vi "Dashboard Main.vi"() -> ()   [LabVIEW 2016]
uses:
  <vilib>/Utility/miscctls.llb/LVRowAndColumnTypeDef.ctl
  <vilib>/event_ctls.llb/eventvkey.ctl
  <vilib>/Rock Robotics/Network Tables/NT Read Numeric Array.vi
  <vilib>/Rock Robotics/Network Tables/NT Read Boolean.vi
  <vilib>/Rock Robotics/Network Tables/NT Write String Array.vi
  <vilib>/Rock Robotics/Network Tables/NT Write Numeric Array.vi
  <vilib>/Rock Robotics/WPI/Dashboard/WPI_DashboardLogging Global.vi
panel:
  out "JS1 Z":dbl(slide) scale=-1.0..1.0 scale format="%#_2e"
  out "JS1 Graph":cluster{"X":dbl, "Y":dbl}[](graph)
  out "JS1 Buttons":T1
  out "JS2 Z":dbl(slide) scale=-1.0..1.0 scale format="%#_2e"
  out "JS2 Graph":cluster{"X":dbl, "Y":dbl}[](graph)
  out "JS2 Buttons":T1
  in  "Camera Settings Right":T2={"Frame Rate"=30, "Compression"=30, "Size"=1, "DB Camera Config"=FALSE} {"Frame Rate" scale=1.0..30.0; "Compression" scale=100.0..-1.0; "Size" items=["640x480", "320x240", "160x120"]}
  in  "Camera Name Right":string(combo)="No Camera Selection"
  out "Camera Info":cluster{"Mbps LED":bool, "Mbps":dbl, "fps":dbl} {"fps" format="%#.1g"; "Mbps" format="%#.1g"}
  in  "Camera Settings":T2={"Frame Rate"=30, "Compression"=30, "Size"=1, "DB Camera Config"=FALSE} {"Frame Rate" scale=1.0..30.0; "Compression" scale=100.0..-1.0; "Size" items=["640x480", "320x240", "160x120"]}
  in  "TCP":refnum<k5>
  in  "Rec Mode":enum32{"Stop", "Record", "Playback"}(radio)
  out "Robot IP":string
  out "Image Message":string="Timeout in Camera Communications"
  in  "Dashboard Tab":T3(tab)
  out "Gyro Angle":dbl
  in  "Refresh Auto":bool
  out "NT Connection":bool
  out "MotorChart R":cluster{"Numeric":dbl, "Numeric":dbl}(graph)
  out "MotorChart L":cluster{"Numeric":dbl, "Numeric":dbl}(graph)
  out "MotorSliders R":cluster{"MotorSlide1":dbl, "MotorSlide2":dbl} {"MotorSlide2" scale=-1.0..1.0 scale format="%#_2e"; "MotorSlide1" scale=-1.0..1.0 scale format="%#_2e"}
  out "MotorSliders L":cluster{"MotorSlide1":dbl, "MotorSlide2":dbl} {"MotorSlide2" scale=-1.0..1.0 scale format="%#_2e"; "MotorSlide1" scale=-1.0..1.0 scale format="%#_2e"}
  out "Gyro":dbl(knob) scale=0.0..360.0
  out "Mode":T4(ring)=enum."Auto Disabled"
  out "Ball Intake Speed":dbl(slide) scale=0.0..1.0
  out "Shooter Speed":dbl(slide) scale=0.0..1.0
  in  "Auto Routines":string(combo)
  out "Auto Cmd":string
  out "Auto Arg":string
  out "Climber":bool
  out "IMU AHRS":cluster{"Pitch":dbl, "Roll":dbl, "Yaw":dbl}
  out "IMU Angle":cluster{"X":dbl, "Y":dbl, "Z":dbl}
  out "Front Left Encoder":dbl
  out "Front Right Encoder":dbl
  out "Back Right Encoder":dbl
  out "Back Left Encoder":dbl
  out "Camera Image Right":T5(plugin-control)
  in  "DB/String 9":string
  in  "DB/String 8":string
  in  "DB/String 7":string
  in  "DB/String 6":string
  in  "DB/String 5":string
  in  "DB/String 4":string
  in  "DB/String 3":string
  in  "DB/String 2":string
  in  "DB/String 1":string
  in  "DB/String 0":string
  in  "DB/Slider 0":dbl(slide) scale=0.0..5.0
  in  "DB/Slider 1":dbl(slide) scale=0.0..5.0
  in  "DB/Slider 2":dbl(slide) scale=0.0..5.0
  in  "DB/Slider 3":dbl(slide) scale=0.0..5.0
  out "DB/LED 3":bool
  out "DB/LED 2":bool
  out "DB/LED 1":bool
  out "DB/LED 0":bool
  in  "DB/Button 3":bool
  in  "DB/Button 2":bool
  in  "DB/Button 1":bool
  in  "DB/Button 0":bool caption="New Name"
  in  "Test Slider":dbl(slide) scale=0.0..100.0 scale format="%#_3g"
  in  "On/Off":bool caption="Solenoid"
  in  "Test Name":u16(ring) items=["Select the test to run..."]
  in  "Test Tree":string(tree)
  in  "Motor":cluster{"Value":dbl, "Enable":bool} {"Value" scale=-1.0..1.0 scale format="%#_3g"}
  out "Progress":T6 {"Test Progress" scale=0.0..100.0}
  in  "Rev/Fwd":cluster{"Forward":bool, "Reverse":bool}
  in  "Test Ring":u16(ring) items=["Monochrome", "Color"]
  out "Cmd Status":string
  in  "Execute Command":bool
  in  "Command Params":string[][](table)
  in  "Command Selection":i32(listbox)
  in  "CheckList":i32(listbox)
  out "Tree":string(tree)
  out "Camera Image":T5(plugin-control)
  out "Background":bool
  in  "Camera Name":string(combo)="No Camera Selection"
  # "Joysticks"
  # "HW"
  # "HW"
  # "Drive Motors"
  # "Front"
  # "Right"
  # "Left"
  # "Back"
  # "This tab is a great place for autonomous settings and robot-specific values.\nPlace controls and indicators inside this tab and match name to\nDashboard Variables on robot. You can also delete this comment."
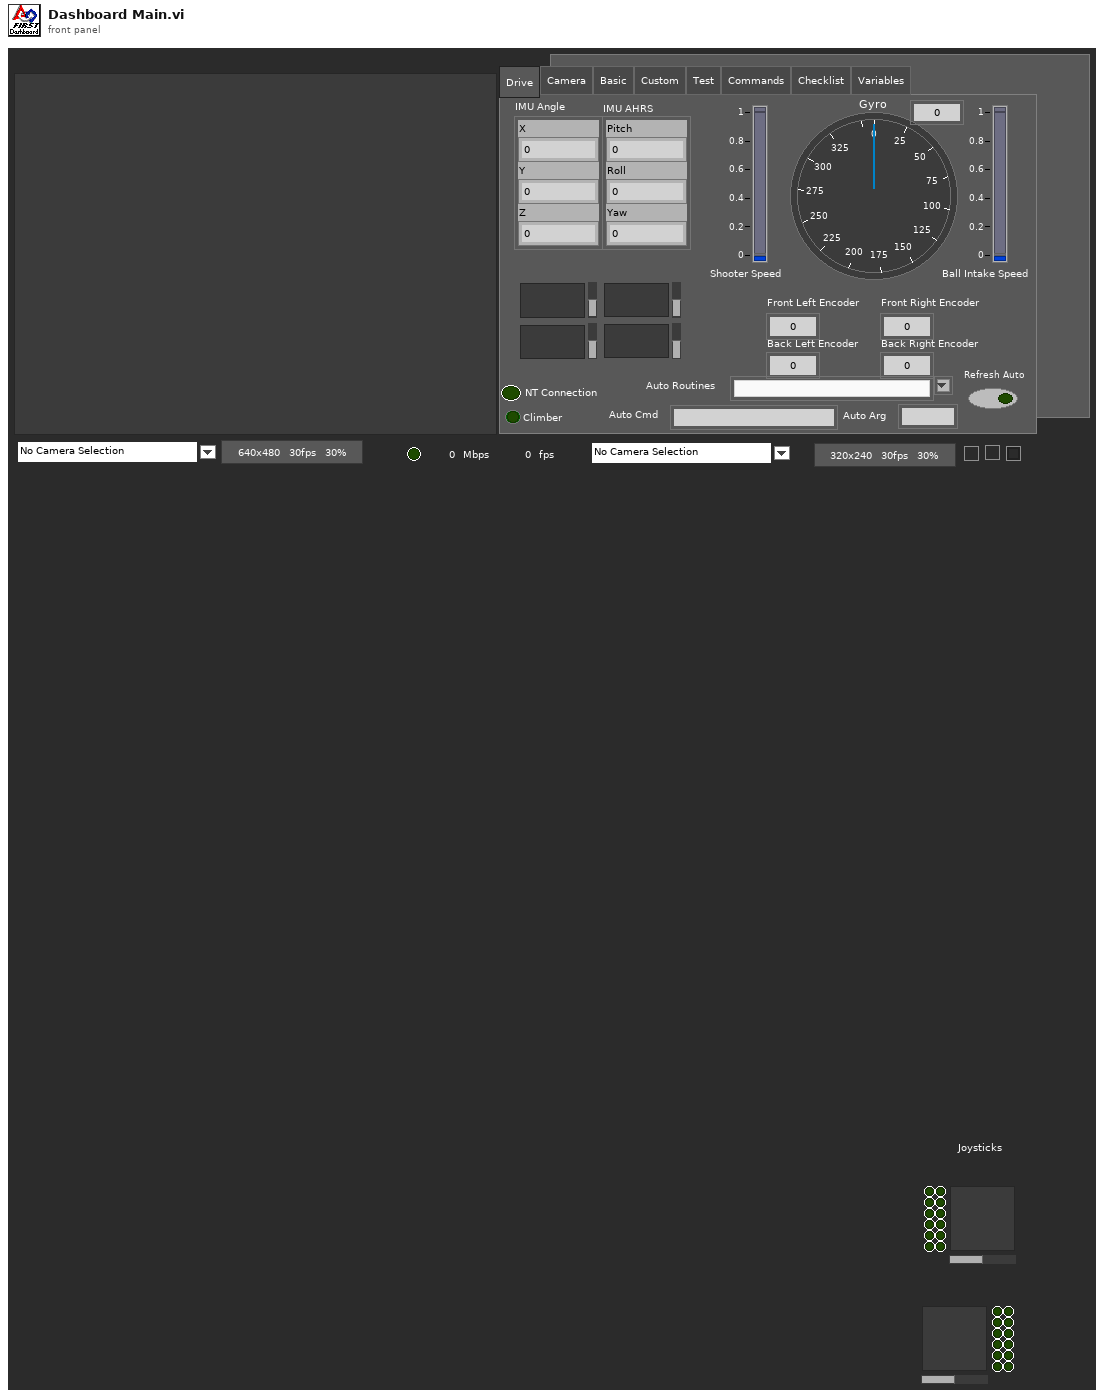
[diagram p1: front panel]
types:
  T1 = cluster{bool, bool, bool, bool, bool, bool, bool, bool, bool, bool, bool, bool}
  T2 = cluster{"Frame Rate":i32, "Compression":i32, "Size":u16, "DB Camera Config":bool}
  T3 = enum32{"Drive", "Camera", "Basic", "Custom", "Test", "Commands", "Checklist", "Variables"}
  T4 = enum8{"Tele-Op Disabled", "Tele-Op Enabled", "Auto Disabled", "Auto Enabled", "Test Disabled", "Test Enabled", "Disconnected", "No Code", "E-Stop"}
  T5 = typedef "IMAQ Image.ctl" = refnum<image>
  T6 = cluster{"Test Progress":u8, "Test Progress Text":string}
  T7 = typedef "Image Type" = u32
  T8 = cluster{"IDs":cluster{"RPC field ID":u16, "Unique ID":u16}, "String":string}
  T9 = enum32{"Drive", "Basic", "Custom", "Test", "Checklist", "Variables"}
  T10 = cluster{"Error Strings":string, "Disable Counts":cluster{u16, u16}, "Rail Faults":cluster{u16, u16, u16}, "Robot IP":string, "DB Mode":u8, "Event Info":cluster{"Name":string, "Type":u8, "Number":u16, "Replay":u8}}
  T11 = cluster{"Storage":cluster{"Disk Free":u64, "RAM Block":u32, "RAM free":u32}, "CPU Utilization":cluster{"CPU % ISR":sgl, "CPU % Time Crit":sgl, "CPU % Timed Str":sgl, "CPU % High":sgl, "CPU % Above":sgl, "CPU % Normal":sgl, "CPU % Low":sgl}, "CAN":cluster{"% Bus Utilization":sgl, "Bus Off Cnt":u32, "TX_FIFO Full Cnt":u32, "Receive Error Cnt":u8, "Transmit Error Cnt":u8}, "HID":cluster{"HID Outputs":u32, "Rumble Low":u16, "Rumble High":u16}[]}
  T12 = cluster{"Status bits":cluster{"Test Mode":bool, "Autonomous":bool, "Enabled":bool, "Code Start":bool, "Brownout":bool, "Reserved 2":bool, "Reserved 3":bool, "E-Stop":bool}, "Code Trace":cluster{"Disabled":bool, "TeleOp":bool, "Auto":bool, "Test":bool}, "Controller Type":enum16{"unknown", "cRIO", "roboRio"}, "Code?":enum16{"unknown", "noCode", "code"}, "Battery V":dbl}
  T13 = cluster{"Control Bits":cluster{"TestMode":bool, "Autonomous":bool, "Enabled":bool, "FMS Present":bool, bool, bool, bool, "E-Stop":bool}, "Team Station ":u8, "Countdown":sgl, "Joystick Values":cluster{"Axes":dbl[], "Buttons":bool[], "POVs":i16[]}[]}
  T14 = cluster{"Axes":dbl[], "Buttons":bool[], "POVs":i16[]}[]
  T15 = cluster{"Numeric Array[0]":dbl, "Numeric Array[1]":dbl, "Numeric Array[2]":dbl, "Numeric Array[3]":dbl, "Numeric Array[4]":dbl, "Numeric Array[5]":dbl, "Numeric Array[6]":dbl, "Numeric Array[7]":dbl, "Numeric Array[8]":dbl}
  T16 = cluster{"Axes":dbl[], "Buttons":bool[], "POVs":i16[]}
  T17 = cluster{"Buttons[0]":bool, "Buttons[1]":bool, "Buttons[2]":bool, "Buttons[3]":bool, "Buttons[4]":bool, "Buttons[5]":bool, "Buttons[6]":bool, "Buttons[7]":bool, "Buttons[8]":bool, "Buttons[9]":bool, "Buttons[10]":bool, "Buttons[11]":bool}
  T18 = cluster{"Camera Image":refnum<vi>, "Dashboard Tab":refnum<vi>, "Background":refnum<vi>, "Rec Mode":refnum<vi>, "Test Slider":refnum<vi>, "On/Off ":refnum<vi>, "Test Ring":refnum<vi>, "Rev/Fwd":refnum<vi>, "Test Name":refnum<vi>, "Motor":refnum<vi>, "Progress":refnum<vi>, "CheckList":refnum<vi>, "Tree":refnum<vi>, "Test Tree":refnum<vi>, "Command Params":refnum<vi>, "Command Selection":refnum<vi>, "Execute Command":refnum<vi>, "Cmd Status":refnum<vi>, "Camera Settings":refnum<vi>, "Camera Name":refnum<vi>, "Camera Info":refnum<vi>, "Camera Settings Right":refnum<vi>, "Camera Name Right":refnum<vi>, "Camera Image Right":refnum<vi>}
  T19 = cluster{"Operation":enum16{"Update", "Clear"}, "Color Box":u32}[]
  T20 = typedef "eventvkey.ctl" = enum16{"ASCII", "Enter", "Return", "Shift", "Ctrl", "Alt", "Cmd", "Opt", "Caps", "NumLock", "Clear", "Break", "Up", "Down", "Left", "Right", "Insert", "Delete", "Home", "End", "PageUp", "PageDown", "Escape", "Help", "Pause", "ScrollLock", "F1", "F2", "F3", "F4", "F5", "F6", "F7", "F8", "F9", "F10", "F11", "F12", "F13", "F14", "F15", "F16", "F17", "F18", "F19", "F20", "F21", "F22", "F23", "F24", "Play", "VolumeUp", "VolumeDown", "Mute", "Two Byte Char"}
  T21 = cluster{"Image Size":bool, "Image Type":bool, "Pixel Value":bool, "ROI Information":bool, "Zoom Factor":bool}
  T22 = cluster{"Operation":enum16{"Update", "Clear"}, "Color Box":u32}
  T23 = typedef "LVRowAndColumnTypeDef.ctl" = cluster{"Row":i32, "Column":i32}
  T24 = cluster{"Shift":bool, "Ctrl":bool, "Alt":bool, "Cmd":bool, "Opt":bool}
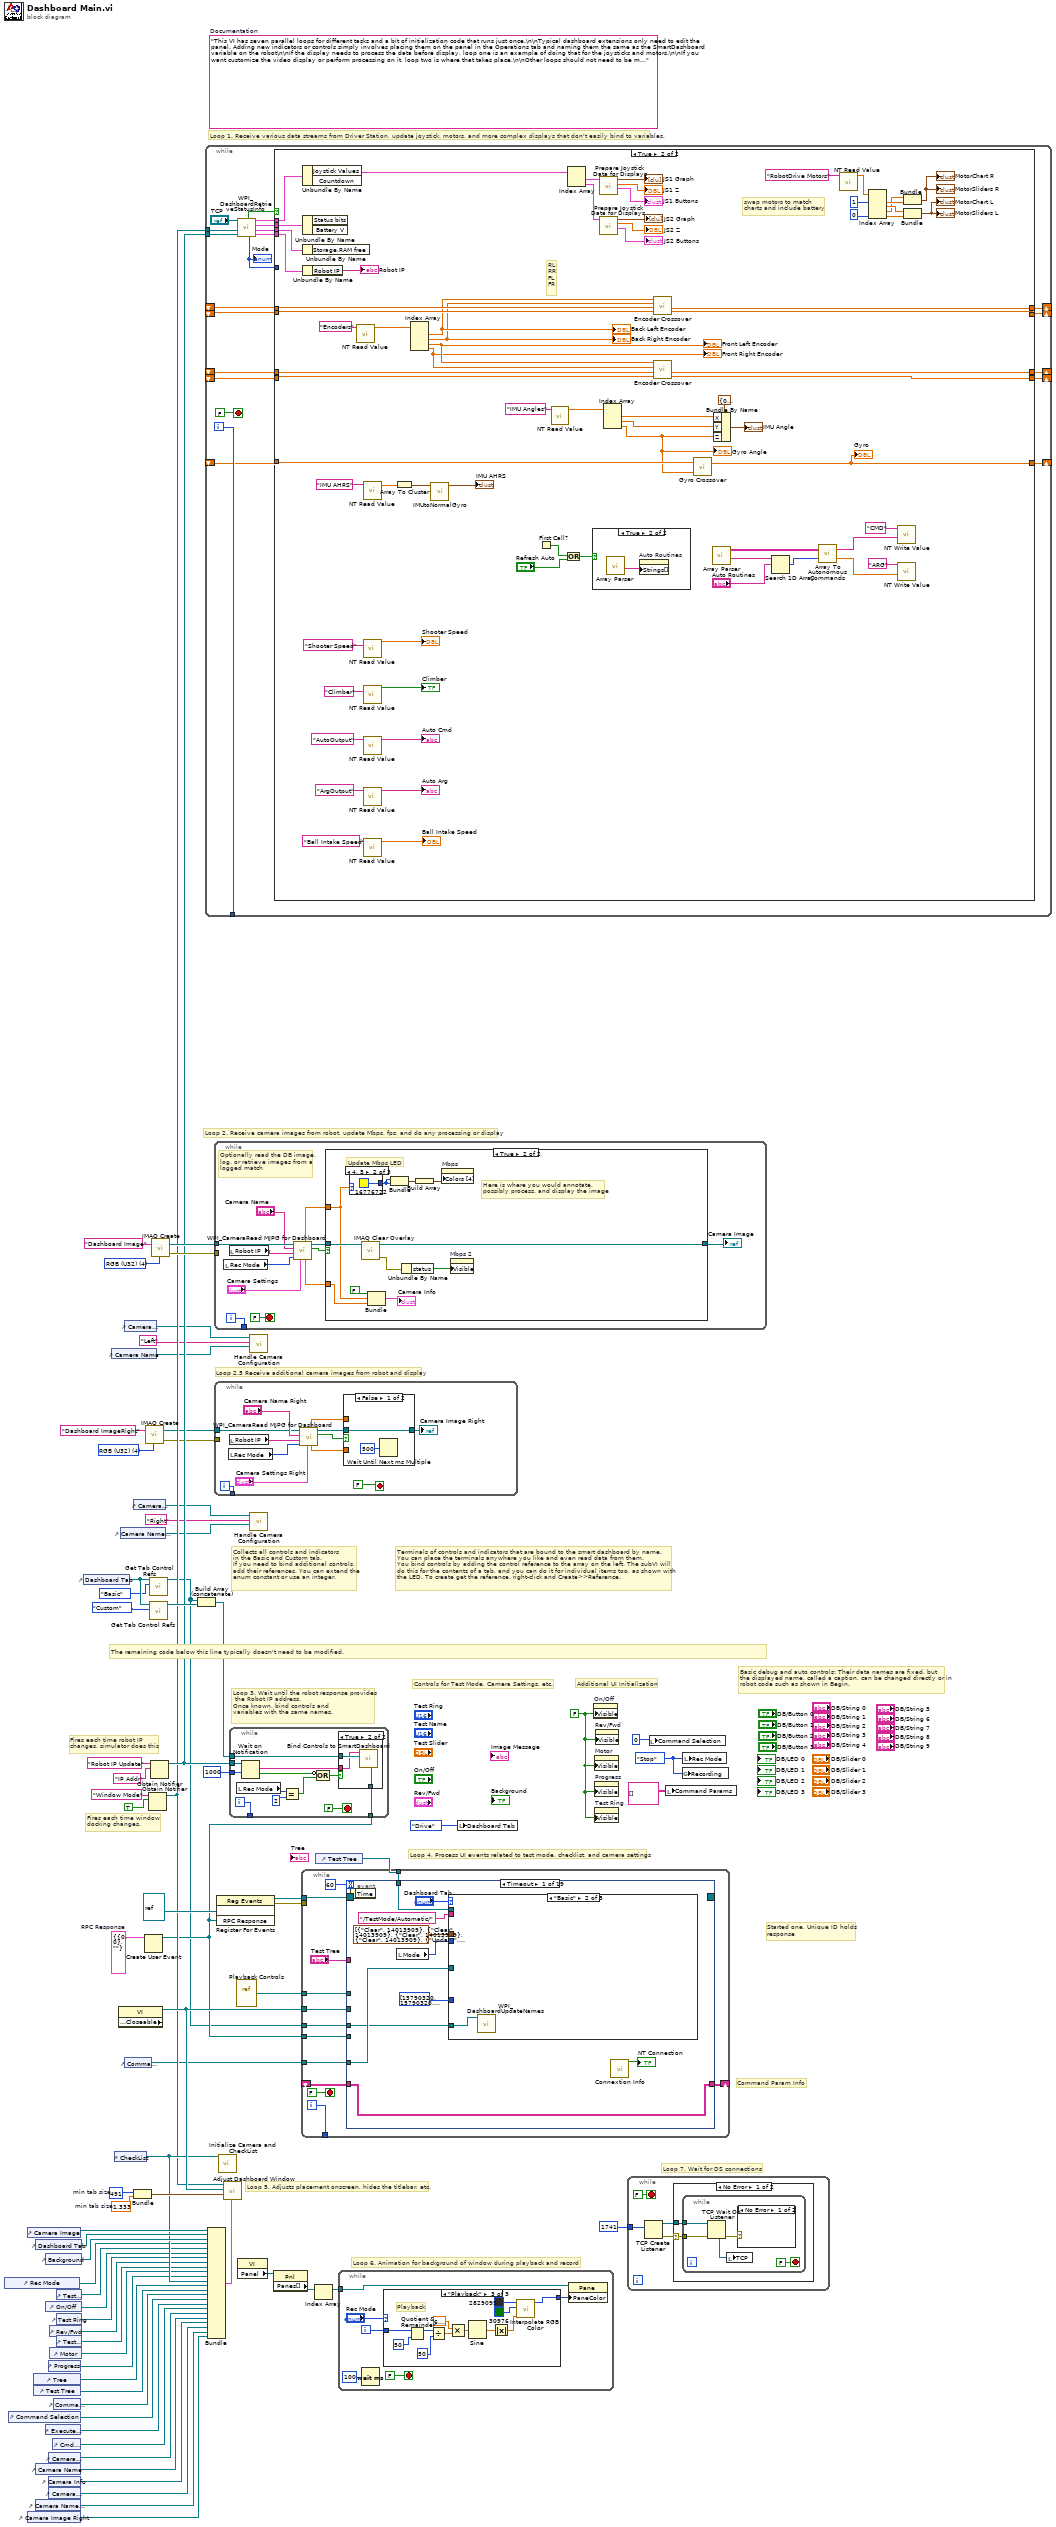
[diagram p0: block diagram]
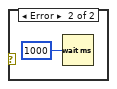
[diagram p3: hidden frame]
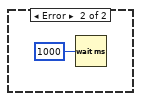
[diagram p4: hidden frame]
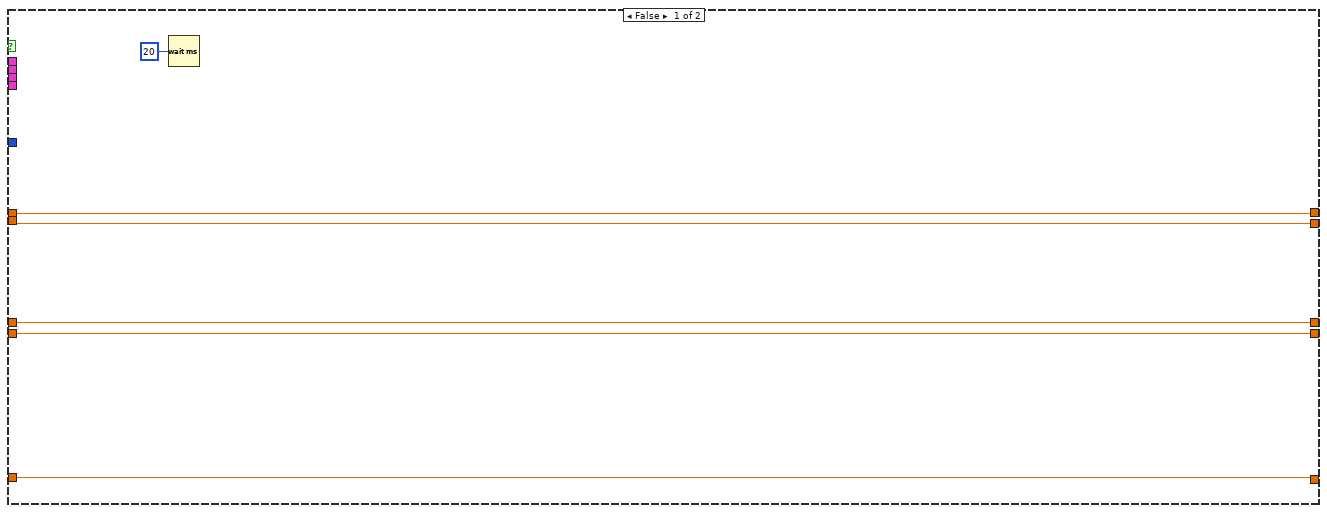
[diagram p5: hidden frame]
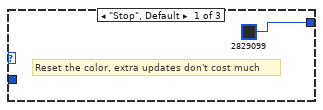
[diagram p7: hidden frame]
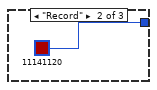
[diagram p8: hidden frame]
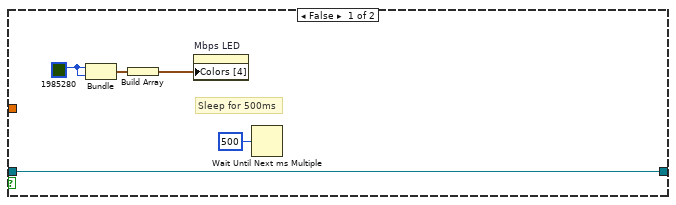
[diagram p10: hidden frame]
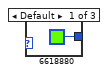
[diagram p11: hidden frame]
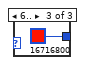
[diagram p12: hidden frame]
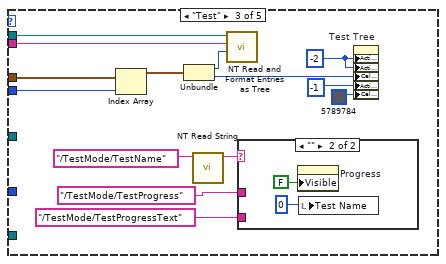
[diagram p14: hidden frame]
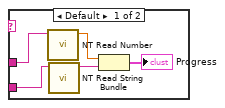
[diagram p15: hidden frame]
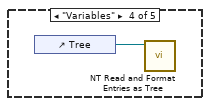
[diagram p16: hidden frame]
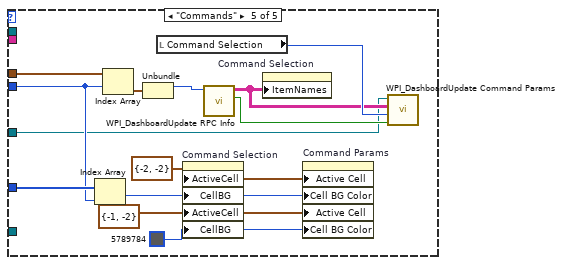
[diagram p17: hidden frame]
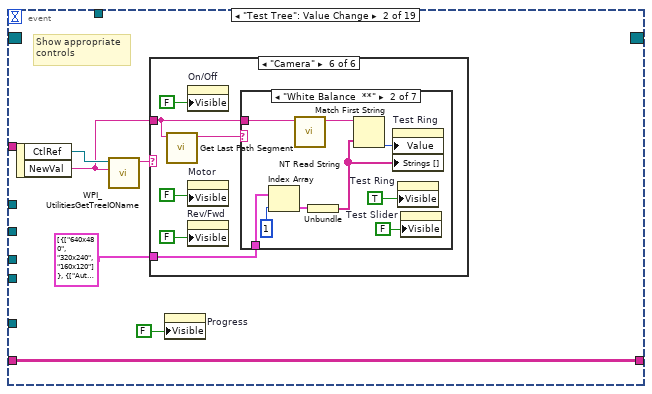
[diagram p18: hidden frame]
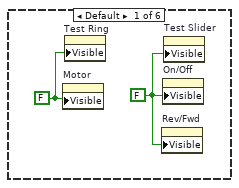
[diagram p19: hidden frame]
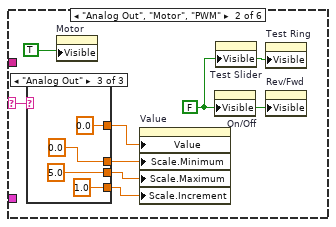
[diagram p20: hidden frame]
diagram:
  w10 = T7 4 items=["Grayscale (U8)", "Grayscale (I16)", "Grayscale (SGL)", "Complex (CSG)", "RGB (U32)", "HSL (U32)", "RGB (U64)"] ("Image Type")
  w24 = T8 {"IDs"={"RPC field ID"=0, "Unique ID"=0}, "String"=""}  # RPC Response
  w49 = 491  # min tab size
  w48 = 1.333  # min tab size
  w56 = enum32{"Stop", "Record", "Playback"}."Stop" ("Rec Mode")
  w31 = FALSE ("Visible")
  (unwired) "This VI has seven parallel loops for different tasks and a bit of initialization code that runs just once.\n\nTypical dashboard extensions only need to edit the panel. Adding new indicators or controls simply involves placing them on the panel in the Operations tab and naming them the same as the SmartDashboard variable on the robot\n\nIf the display needs to process the data before display, loop one is an example of doing that for the joysticks and motors.\n\nIf you want customize the video display or perform processing on it, loop two is where that takes place.\n\nOther loops should not need to be modified. They are pretty standard, and document the task they perform."  # Documentation
  w73 = T7 4 items=["Grayscale (U8)", "Grayscale (I16)", "Grayscale (SGL)", "Complex (CSG)", "RGB (U32)", "HSL (U32)", "RGB (U64)"] ("Image Type")
  # "Loop 2.5 Receive additional camera images from robot and display"
  # "Command Param Info"
  # "Started one, Unique ID holds\nresponse"
  # "Loop 7. Wait for DS connections"
  # "Basic debug and auto controls: Their data names are fixed, but\nthe displayed name, called a caption, can be changed directly or in\nrobot code such as shown in Begin."
  # "Controls for Test Mode, Camera Settings, etc."
  # "Additional UI Initialization"
  # "Loop 6. Animation for background of window during playback and record"
  # "Fires each time robot IP\nchanges, simulator does this"
  # "Fires each time window\ndocking changes."
  # "Collects all controls and indicators\nin the Basic and Custom tab.\nIf you need to bind additional controls,\nadd their references. You can extend the\nenum constant or use an integer."
  # "The remaining code below this line typically doesn't need to be modified."
  # "Loop 4. Process UI events related to test mode, checklist, and camera settings"
  # "Terminals of controls and indicators that are bound to the smart dashboard by name.\nYou can place the terminals anywhere you like and even read data from them.\nYou bind controls by adding the control reference to the array on the left. The subVI will\ndo this for the contents of a tab, and you can do it for individual items too, as shown with\nthe LED. To create get the reference, right-click and Create>>Reference."
  # "Loop 3. Wait until the robot response provides\n the Robot IP address.\nOnce known, bind controls and\nvariables with the same names."
  # "Loop 5. Adjusts placement onscreen, hides the titlebar, etc."
  # "Loop 1. Receive various data streams from Driver Station, update joystick, motors, and more complex displays that don't easily bind to variables."
  # "Loop 2. Receive camera images from robot, update Mbps, fps, and do any processing or display"
  n1 = control-ref of="Rec Mode"() -> (w37:refnum<vi>)
  n2 = control-ref of="Command Selection"() -> (w23:refnum<vi>)
  n3 = control-ref of="Camera Image Right"() -> (w1:refnum<vi>)
  n4 = control-ref of="Camera Image"() -> (w51:refnum<vi>)
  n5 = control-ref of="Tree"() -> (w41:refnum<vi>)
  n6 = control-ref of="Test Tree"() -> (w40:refnum<vi>)
  n7 = control-ref of="Dashboard Tab"() -> (w50:refnum<vi>)
  n8 = control-ref of="Camera Name"() -> (w14:refnum<vi>)
  n9 = control-ref of="Camera Name Right"() -> (w2:refnum<vi>)
  n10 = control-ref of="Execute Command"() -> (w25:refnum<vi>)
  n11 = control-ref of="Background"() -> (w46:refnum<vi>)
  n12 = control-ref of="On/Off"() -> (w35:refnum<vi>)
  n13 = control-ref of="Progress"() -> (w32:refnum<vi>)
  n14 = control-ref of="Camera Settings"() -> (w15:refnum<vi>)
  n15 = control-ref of="Camera Info"() -> (w13:refnum<vi>)
  n16 = control-ref of="Camera Settings Right"() -> (w3:refnum<vi>)
  n17 = control-ref of="Rev/Fwd"() -> (w33:refnum<vi>)
  n18 = control-ref of="Motor"() -> (w38:refnum<vi>)
  n19 = control-ref of="Cmd Status"() -> (w19:refnum<vi>)
  n20 = control-ref of="Command Params"() -> (w26:refnum<vi>)
  n21 = control-ref of="Test Slider"() -> (w36:refnum<vi>)
  n22 = control-ref of="Test Ring"() -> (w34:refnum<vi>)
  n23 = control-ref of="Test Name"() -> (w39:refnum<vi>)
  n24 = control-ref of="Dashboard Tab"() -> (w54:refnum<vi>)
  n25 = control-ref of="Camera Name"() -> (w16:refnum<vi>)
  n26 = control-ref of="CheckList"() -> (w42:refnum<vi>)
  n27 = property class="VI" props=["Front Panel.Closeable"]() -> (reference out=w55:refnum<vi>)  [unwired: 2 in, 2 out]
  n28 = control-ref of="Camera Name Right"() -> (w6:refnum<vi>)
  n29 = control-ref of="Camera Settings"() -> (w17:refnum<vi>)
  n30 = control-ref of="Command Params"() -> (w18:refnum<vi>)
  n31 = control-ref of="Camera Settings Right"() -> (w7:refnum<vi>)
  n32 = Bundle("min tab size"=w49, "min tab size"=w48) -> (w47:cluster{"min tab size":i32, "min tab size":dbl})  [unwired: 1 in]
  n33 = Create User Event(user event datatype=w24) -> (user event=w20:refnum<user-event>)  [unwired: 1 in, 1 out]
  n34 = call "IMAQ Create"("Image Name"="Dashboard ImageRight", "Image Type"=w10) -> ("New Image"=w9:T5, "error out"=w8:errorcluster)  [unwired: 2 in, 1 out]
  n35 = Obtain Notifier(name (unnamed)="Window Mode", notification data type=TRUE) -> (notifier out=w29:refnum<notifier>)  [unwired: 2 in, 2 out]
  n36 = call <vilib>:"Get Tab Control Refs.vi"("Page Index"=T9."Basic" ("Dashboard Tab"), "TabControl in"=w54) -> ("ControlsOnPage"=w12:refnum<vi>[])  [unwired: 9 in]
  n37 = call <vilib>:"Get Tab Control Refs.vi"("Page Index"=T9."Custom" ("Dashboard Tab"), "TabControl in"=w54) -> ("ControlsOnPage"=w53:refnum<vi>[])  [unwired: 9 in]
  n38 = Obtain Notifier(name (unnamed)="Robot IP Update", notification data type="IP Addr" ("name (unnamed)")) -> (notifier out=w30:refnum<notifier>)  [unwired: 2 in, 2 out]
  n39 = call "IMAQ Create"("Image Name"="Dashboard Image", "Image Type"=w73) -> ("New Image"=w71:T5, "error out"=w70:errorcluster)  [unwired: 2 in, 1 out]
  n40 = Build Array (concatenate)(w12, w53) -> (w52:refnum<vi>[])
  n41 = while {
    tunnel: [w93] -> _
    tunnel: w30 -> [w87]
    tunnel: w29 -> [w84]
    shift-right: [w82] -> _
    shift-left: _ -> [w83]
    shift-right: [w80] -> _
    shift-left: _ -> [w81]
    shift-right: [w78] -> _
    shift-left: _ -> [w79]
    shift-right: [w74] -> _
    shift-left: _ -> [w75]
    shift-right: [w76] -> _
    shift-left: _ -> [w77]
    i -> [w93]
    stop <- FALSE stop-if-true
    n42 = call <vilib>:"WPI_DashboardRetrieveStatusInfo.vi"("Binding Refnum"=w87, "Window Mode Notifier"=w84, "TCP Cnx"="TCP") -> ("Power and Errors"=w88:T10, "Robot Metrics"=w91:T11, "Status Info"=w92:T12, "Control Info"=w89:T13, "Robot Mode"=w86:T4, "Process?"=w90:bool)  [unwired: 3 in]
    "Mode" <- w86
    n43 = case shown="True" w90 {
      tunnel: w92 -> [_ w172]
      tunnel: w91 -> [_ w171]
      tunnel: w89 -> [_ w170]
      tunnel: w88 -> [_ w169]
      tunnel: w86 -> [_ _]
      tunnel: [w98 w146] -> w82
      tunnel: [w97 w145] -> w80
      tunnel: w83 -> [w98 w144]
      tunnel: w81 -> [w97 w143]
      tunnel: w79 -> [w99 w142]
      tunnel: [w99 w102] -> w78
      tunnel: w77 -> [w96 w110]
      tunnel: [w96 w109] -> w76
      tunnel: w75 -> [w95 w108]
      tunnel: [w95 w107] -> w74
      frame False {
        n44 = Wait (ms)(milliseconds to wait=u32 20) -> ()  [unwired: 1 out]
      }
      frame True {
        # "RL\nRR\nFL\nFR"
        # "swap motors to match\ncharts and include battery"
        n45 = Unbundle By Name(w170) -> ("Joystick Values"=w160:T14)  [unwired: 1 out]
        n46 = Unbundle By Name(w172) -> ()  [unwired: 2 out]
        n47 = Unbundle By Name(w171) -> ()  [unwired: 1 out]
        n48 = Unbundle By Name(w169) -> ("Robot IP"=→"Robot IP":string)
        n49 = call-poly <vilib>:"NT Read Value.vi"("Name"="Encoders") -> ("Numeric Array"=w148:dbl[])  [unwired: 9 in, 1 out]
        n50 = call-poly <vilib>:"NT Read Value.vi"("Name"="Shooter Speed") -> ("Numeric"=→"Shooter Speed":dbl)  [unwired: 9 in, 1 out]
        n51 = call-poly <vilib>:"NT Read Value.vi"("Name"="Climber") -> ("Boolean"=→"Climber":bool)  [unwired: 9 in, 1 out]
        n52 = call-poly <vilib>:"NT Read Value.vi"("Name"="AutoOutput") -> ("String"=→"Auto Cmd":string)  [unwired: 9 in, 1 out]
        n53 = call-poly <vilib>:"NT Read Value.vi"("Name"="ArgOutput") -> ("String"=→"Auto Arg":string)  [unwired: 9 in, 1 out]
        n54 = call-poly <vilib>:"NT Read Value.vi"("Name"="IMU AHRS") -> ("Numeric Array"=w114:dbl[])  [unwired: 9 in, 1 out]
        n55 = call-poly <vilib>:"NT Read Value.vi"("Name"="Ball Intake Speed") -> ("Numeric"=→"Ball Intake Speed":dbl)  [unwired: 9 in, 1 out]
        n56 = Array To Cluster(array=w114) -> (cluster=w112:T15)
        n57 = Index Array(array=w148) -> (element #1=w106:dbl, element #2=w105:dbl, element #3=w104:dbl, element #4=w103:dbl)  [unwired: 4 in]
        "Front Left Encoder" <- w104
        "Front Right Encoder" <- w103
        "Back Left Encoder" <- w106
        "Back Right Encoder" <- w105
        n58 = call "IMUtoNormalGyro.vi"("IMU Data"=w112) -> ("IMU Data Out"=→"IMU AHRS":cluster{"Pitch":dbl, "Roll":dbl, "Yaw":dbl})  [unwired: 5 in, 3 out]
        n59 = First Call?() -> (First Call?: T/F=w133:bool)
        n60 = call-poly <vilib>:"NT Read Value.vi"("Name"="IMU Angles") -> ("Numeric Array"=w119:dbl[])  [unwired: 9 in, 1 out]
        n61 = Or(x=w133, y="Refresh Auto") -> (x .or. y?=w132:bool)
        n62 = Index Array(array=w160) -> (element #1=w159:T16, element #2=w155:T16)  [unwired: 2 in]
        n63 = case shown="True" w132 {
          frame False {
          }
          frame True {
            n64 = call "Array Parser.vi"() -> ("Auto Routines"=w173:string[])  [unwired: 9 in, 2 out]
            n65 = property on="Auto Routines" class="CmbBox"("Strings[]"=w173) -> ()  [unwired: 2 in, 2 out]
          }
        }
        n66 = call "Prepare Joystick Data for Displays.vi"("Joystick Values"=w155) -> ("Buttons"=→"JS2 Buttons":T17, "Z Axis"=→"JS2 Z":dbl, "Cartesian Data"=→"JS2 Graph":cluster{"X axis":dbl, "X axis":dbl}[])  [unwired: 8 in]
        n67 = call "Prepare Joystick Data for Displays.vi"("Joystick Values"=w159) -> ("Buttons"=→"JS1 Buttons":T17, "Z Axis"=→"JS1 Z":dbl, "Cartesian Data"=→"JS1 Graph":cluster{"X axis":dbl, "X axis":dbl}[])  [unwired: 8 in]
        n68 = Index Array(array=w119) -> (element #1=w117:dbl, element #2=w116:dbl, element #3=w101:dbl)  [unwired: 3 in]
        "Gyro Angle" <- w101
        n69 = call "Encoder Crossover.vi"("Previous Value 2"=w108, "Previous Value"=w110, "Encoder Value 2"=w105, "Encoder Value"=w106) -> ("Encoder Output 2"=w107:dbl, "Encoder Output"=w109:dbl)  [unwired: 2 in]
        n70 = call "Encoder Crossover.vi"("Previous Value 2"=w143, "Previous Value"=w144, "Encoder Value 2"=w103, "Encoder Value"=w104) -> ("Encoder Output 2"=w145:dbl, "Encoder Output"=w146:dbl)  [unwired: 2 in]
        n71 = call "Gyro Crossover.vi"("Gyro Value"=w101, "Previous Value"=w142) -> ("Gyro Value"=w102:dbl)
        "Gyro" <- w102
        n72 = call "Array Parser.vi"() -> ("Auto Routines"=w136:string[], "CSV Data"=w134:string[][][])  [unwired: 9 in, 1 out]
        n73 = Bundle By Name(cluster=cluster{"X":dbl, "Y":dbl, "Z":dbl} {"X"=0.0, "Y"=0.0, "Z"=0.0} ("IMU Angles"), "X"=w117, "Y"=w116, "Z"=w101) -> (→"IMU Angle":cluster{"X":dbl, "Y":dbl, "Z":dbl})
        n74 = Search 1D Array(1D array=w136, element="Auto Routines") -> (index of element=w135:i32)  [unwired: 1 in]
        n75 = call "Array To Autonomous Commands.vi"("Which"=w135, "Input Array"=w134) -> ("Float Output Array"=w138:dbl[], "String Output Array"=w139:string[])
        n76 = call-poly <vilib>:"NT Read Value.vi"("Name"="RobotDrive Motors") -> ("Numeric Array"=w150:dbl[])  [unwired: 9 in, 1 out]
        n77 = Index Array(array=w150, index #1=1, index #4=0) -> (element #1=w164:dbl, element #2=w165:dbl, element #3=w163:dbl, element #4=w168:dbl)  [unwired: 2 in]
        n78 = call-poly <vilib>:"NT Write Value.vi"("String Array"=w139, "Name"="CMD") -> ()  [unwired: 9 in, 1 out]
        n79 = call-poly <vilib>:"NT Write Value.vi"("Numeric Array"=w138, "Name"="ARG") -> ()  [unwired: 9 in, 1 out]
        n80 = Bundle("Numeric"=w163, "Numeric"=w164) -> (→"MotorChart R" →"MotorSliders R":cluster{"Numeric":dbl, "Numeric":dbl})  [unwired: 1 in]
        n81 = Bundle("Numeric"=w165, "Numeric"=w168) -> (→"MotorChart L" →"MotorSliders L":cluster{"Numeric":dbl, "Numeric":dbl})  [unwired: 1 in]
      }
    }
  }
  n82 = Bundle("Camera Image"=w51, "Dashboard Tab"=w50, "Background"=w46, "Rec Mode"=w37, "Test Slider"=w36, "On/Off"=w35, "Test Ring"=w34, "Rev/Fwd"=w33, "Test Name"=w39, "Motor"=w38, "Progress"=w32, "CheckList"=w42, "Tree"=w41, "Test Tree"=w40, "Command Params"=w26, "Command Selection"=w23, "Execute Command"=w25, "Cmd Status"=w19, "Camera Settings"=w15, "Camera Name"=w14, "Camera Info"=w13, "Camera Settings Right"=w3, "Camera Name Right"=w2, "Camera Image Right"=w1) -> (w43:T18)  [unwired: 1 in]
  n83 = while {
    tunnel: w71 -> [w183]
    tunnel: w70 -> [_]
    tunnel: [w184] -> _
    i -> [w184]
    stop <- FALSE stop-if-true
    # "Optionally read the DB image,\nlog, or retrieve images from a\nlogged match"
    n84 = local read "Rec Mode"() -> (w179:enum32{"Stop", "Record", "Playback"})
    n85 = local read "Robot IP"() -> (w178:string)
    n86 = call <vilib>:"WPI_CameraRead MJPG for Dashboard.vi"("Camera Settings"="Camera Settings", "Rec Mode"=w179, "Robot IP"=w178, "Camera Name"="Camera Name", "Refnum in"=w183) -> ("Active"=w181:bool, "Refnum out"=w182:T5, "FPS"=w180:dbl, "Bandwidth (Mbps)"=w177:dbl)  [unwired: 3 in]
    n87 = case shown="True" w181 {
      tunnel: w182 -> [w186 w197]
      tunnel: w177 -> [_ w194]
      tunnel: w180 -> [_ w195]
      tunnel: [w186 w191] -> w174
      frame False {
        w188 = u32 1985280 ("Color Box")
        # "Sleep for 500ms"
        n88 = Bundle("Color Box"=w188, "Color Box"=w188) -> (w189:cluster{"Color Box":u32, "Color Box":u32})  [unwired: 1 out]
        n89 = Build Array(w189) -> (w187:cluster{"Color Box":u32, "Color Box":u32}[])
        n90 = property on="Mbps LED" class="Bool (strict)"("Colors [4]"=w187) -> ()  [unwired: 2 in, 2 out]
        n91 = Wait Until Next ms Multiple(millisecond multiple=u32 500) -> ()  [unwired: 1 out]
      }
      frame True {
        # "Here is where you would annotate,\npossibly process, and display the image"
        # "Update Mbps LED"
        n92 = case shown="4, 5" w194 {
          tunnel: [u32 6618880 ("Color Box") u32 16776722 ("Color Box") u32 16716800 ("Color Box")] -> w198
          frame Default {
          }
          frame 4, 5 {
          }
          frame 6.. {
          }
        }
        n93 = call "IMAQ Clear Overlay"("Image"=w197) -> ("error out"=w200:errorcluster, "Image Out"=w191:T5)  [unwired: 2 in, 7 out]
        n94 = Bundle(FALSE, "Bandwidth (Mbps)"=w194, "FPS"=w195) -> (→"Camera Info":cluster{bool, "Bandwidth (Mbps)":dbl, "FPS":dbl})  [unwired: 1 in]
        n95 = Bundle("Color Box"=w198, "Color Box"=w198) -> (w199:cluster{"Color Box":u32, "Color Box":u32})  [unwired: 1 out]
        n96 = Unbundle By Name(w200) -> ("status"=w201:bool)
        n97 = Build Array(w199) -> (w196:cluster{"Color Box":u32, "Color Box":u32}[])
        n98 = property on="Mbps" class="Bool (strict)"("Colors [4]"=w196) -> ()  [unwired: 2 in, 2 out]
        n99 = property on="Mbps 2" class="Str"("Visible"=w201) -> ()  [unwired: 2 in, 2 out]
      }
    }
    "Camera Image" <- w174
  }
  n100 = while {
    tunnel: w9 -> [w215]
    tunnel: w8 -> [_]
    tunnel: [w209] -> _
    i -> [w209]
    stop <- FALSE stop-if-true
    n101 = local read "Rec Mode"() -> (w213:enum32{"Stop", "Record", "Playback"})
    n102 = local read "Robot IP"() -> (w214:string)
    n103 = call <vilib>:"WPI_CameraRead MJPG for Dashboard.vi"("Camera Settings"="Camera Settings Right", "Rec Mode"=w213, "Robot IP"=w214, "Camera Name"="Camera Name Right", "Refnum in"=w215) -> ("Active"=w208:bool, "Refnum out"=w211:T5, "FPS"=w206:dbl, "Bandwidth (Mbps)"=w207:dbl)  [unwired: 3 in]
    n104 = case shown="False" w208 {
      tunnel: w211 -> [w217 w219]
      tunnel: w207 -> [_ _]
      tunnel: w206 -> [_ _]
      tunnel: [w217 w219] -> w205
      frame False {
        n105 = Wait Until Next ms Multiple(millisecond multiple=u32 500) -> ()  [unwired: 1 out]
      }
      frame True {
      }
    }
    "Camera Image Right" <- w205
  }
  n106 = register-events(refnum<vi> refnum, w20) -> (reference out=w60:refnum<event-registration>, error out=w59:errorcluster)  [unwired: 2 in]
  n107 = call "Initialize Camera and CheckList.vi"("ListBox in"=w42) -> ()  [unwired: 11 in]
  n108 = call "Adjust Dashboard Window.vi"("Sizing Refnums"=w43, "Size Constraints"=w47, "VI"=w55, "WIn Mode"=w29) -> ()  [unwired: 8 in]
  n109 = while {
    tunnel: w52 -> [w231]
    tunnel: w30 -> [w229]
    tunnel: [w227] -> _
    tunnel: u32 1000 ("milliseconds to wait") -> [w226]
    tunnel: w20 -> [w220]
    i -> [w227]
    stop <- FALSE stop-if-true
    n110 = local read "Rec Mode"() -> (w222:enum32{"Stop", "Record", "Playback"})
    n111 = Wait on Notification(notifier=w229, timeout in ms (-1)=w226) -> (notification=w228:string, timed out?=w224:bool)  [unwired: 2 in, 2 out]
    n112 = Equal?(x=w222, y=u16 2 ("Rec Mode")) -> (x = y?=w223:bool)
    n113 = Compound Arithmetic op=OR(invert w224, w223) -> (w225:bool)
    n114 = case shown="True" w225 {
      tunnel: w231 -> [_ w234]
      tunnel: w228 -> [_ w233]
      tunnel: w220 -> [_ w232]
      frame False {
      }
      frame True {
        n115 = call <vilib>:"Bind Controls to SmartDashboard.vi"("RPC ref"=w232, "Bound Control Refs"=w234, "Server IP Address"=w233) -> ()  [unwired: 9 in]
      }
    }
  }
  n116 = vi-ref "Playback Controls.vi"() -> (w61:refnum<vi>)
  n117 = property class="VI"() -> ("Panel"=w63:refnum<vi>)  [unwired: 2 in, 2 out]
  n118 = call "Handle Camera Configuration.vi"("CameraNameRef"=w16, "Camera File Name"="Left", "ClusterRef"=w17) -> ()  [unwired: 9 in]
  n119 = call "Handle Camera Configuration.vi"("CameraNameRef"=w6, "Camera File Name"="Right", "ClusterRef"=w7) -> ()  [unwired: 9 in]
  n120 = property class="Pnl"(reference=w63) -> ("Panes[]"=w64:refnum<vi>[])  [unwired: 1 in, 2 out]
  n121 = Index Array(array=w64) -> (element=w62:refnum<vi>)  [unwired: 1 in]
  n122 = control-ref of="Test Tree"() -> (w65:refnum<vi>)
  n123 = while {
    tunnel: [w244] -> _
    tunnel: w65 -> [w243]
    tunnel: w61 -> [w242]
    tunnel: w60 -> [w241]
    tunnel: w59 -> [_]
    tunnel: w55 -> [w240]
    tunnel: w20 -> [w239]
    tunnel: w18 -> [w238]
    shift-right: [w237] -> _
    shift-left: _ -> [w236]
    tunnel: w12 -> [w235]
    i -> [w244]
    stop <- FALSE stop-if-true
    n124 = event shown="[0] Timeout" {
      selector: w241 -> [_ _ _ _ _ _ _ _ _ _ _ _ _ _ _ _ _ _ _]
      dyn-events: [_ _ _ _ _ _ _ _ _ _ _ _ _ _ w494 _ _ _ _] -> _
      timeout: u32 60 ("milliseconds to wait") -> [_ _ _ _ _ _ _ _ _ _ _ _ _ _ _ _ _ _ _]
      tunnel: w243 -> [w256 _ _ _ _ _ _ _ _ _ _ _ _ _ _ _ _ _ _]
      tunnel: "Test Tree" -> [_ _ _ _ _ _ _ _ _ w461 w469 w471 w475 w483 _ _ _ _ _]
      tunnel: w242 -> [_ _ _ _ _ _ _ _ _ _ _ _ _ _ w496 _ w514 _ _]
      tunnel: w240 -> [_ _ _ _ _ _ _ _ _ _ _ _ _ _ w492 _ _ _ _]
      tunnel: w239 -> [_ _ _ _ _ _ _ _ _ _ _ _ _ _ w488 _ _ _ _]
      tunnel: w238 -> [w251 _ _ _ w412 _ _ _ _ _ _ _ _ _ _ _ _ _ _]
      tunnel: [w250 w295 w397 w402 w410 w419 w429 w436 w448 w460 w467 w470 w474 w482 w487 w509 w511 w515 w526] -> w237
      tunnel: w236 -> [w250 w295 w397 w402 w410 _ _ w436 w448 w460 w467 w470 w474 w482 w487 w509 w511 w515 w526]
      tunnel: w235 -> [w248 _ _ _ _ _ _ _ _ _ _ _ _ _ _ _ _ _ _]
      event Timeout {
        n125 = event-data() -> ()  [unwired: 1 in, 1 out]
        n126 = local read "Mode"() -> (w253:T4)
        n127 = case shown="\"Basic\"" "Dashboard Tab" {
          tunnel: w256 -> [_ _ w272 _ _]
          tunnel: "/TestMode/Automatic/" ("Name Pattern") -> [_ _ w271 _ _]
          tunnel: T19 [{"Operation"=enum."Clear", "Color Box"=14013909}, {"Operation"=enum."Clear", "Color Box"=14013909}, {"Operation"=enum."Clear", "Color Box"=14013909}, {"Operation"=enum."Clear", "Color Box"=14013909}, {"Operation"=enum."Update", "Color Box"=14013909}, {"Operation"=enum."Update", "Color Box"=16777215}, {"Operation"=enum."Clear", "Color Box"=14013909}, {"Operation"=enum."Clear", "Color Box"=14013909}, {"Operation"=enum."Clear", "Color Box"=14013909}] -> [_ _ w264 _ w288]
          tunnel: w253 -> [_ _ w263 _ w287]
          tunnel: u32[] [15790320, 15790320, 15790320, 15790320, 16777215, 16777215, 15790320, 15790320, 15790320] -> [_ _ _ _ w293]
          tunnel: w251 -> [_ _ _ _ w281]
          tunnel: w248 -> [_ w258 _ _ _]
          frame "Custom", Default {
          }
          frame "Basic" {
            n128 = call <vilib>:"WPI_DashboardUpdateNames.vi"("Controls on Tab"=w258) -> ()  [unwired: 11 in]
          }
          frame "Test" {
            w270 = -2 ("Active Item:Row Number")
            n129 = Index Array(array=w264, index=w263) -> (element=w265:T22)
            n130 = Unbundle(w265) -> ("Operation"=w266:enum16{"Update", "Clear"}, "Color Box"=w267:u32)
            n131 = call <vilib>:"NT Read String.vi"("Name"="/TestMode/TestName") -> ("String"=w261:string)  [unwired: 9 in, 1 out]
            n132 = call <vilib>:"NT Read and Format Entries as Tree.vi"("Operation"=w266, "Name Pattern"=w271, "Tree Refnum"=w272) -> ()  [unwired: 7 in, 2 out]
            n133 = case shown="\"\"" w261 {
              tunnel: "/TestMode/TestProgress" ("Name") -> [w274 _]
              tunnel: "/TestMode/TestProgressText" ("Name") -> [w273 _]
              frame Default {
                n134 = call <vilib>:"NT Read Number.vi"("Name"=w274) -> ("Numeric"=w275:dbl)  [unwired: 9 in, 1 out]
                n135 = call <vilib>:"NT Read String.vi"("Name"=w273) -> ("String"=w276:string)  [unwired: 9 in, 1 out]
                n136 = Bundle("Numeric"=w275, "String"=w276) -> (→"Progress":cluster{"Numeric":dbl, "String":string})  [unwired: 1 in]
              }
              frame "" {
                n137 = property on="Progress" class="Clust (strict)"("Visible"=FALSE) -> ()  [unwired: 2 in, 2 out]
                n138 = local write "Test Name"(u16 0) -> ()
              }
            }
            n139 = property on="Test Tree" class="Tree (strict)"("Active Item Row Number"=w270, "ActiveColNum"=w270, "CellBG"=w267, "Active Item Row Number"=-1 ("Active Item:Row Number"), "CellBG"=u32 5789784 ("Color Box")) -> ()  [unwired: 2 in, 2 out]
          }
          frame "Variables" {
            n140 = control-ref of="Tree"() -> (w280:refnum<vi>)
            n141 = call <vilib>:"NT Read and Format Entries as Tree.vi"("Tree Refnum"=w280) -> ()  [unwired: 9 in, 2 out]
          }
          frame "Commands" {
            w289 = u32 5789784 ("Color Box")
            w290 = T23 {"Row"=-1, "Column"=-2} ("Active Cell:Active Cell")
            w292 = T23 {"Row"=-2, "Column"=-2} ("Active Cell:Active Cell")
            n142 = Index Array(array=w293, index=w287) -> (element=w291:u32)
            n143 = Index Array(array=w288, index=w287) -> (element=w286:T22)
            n144 = Unbundle(w286) -> ("Operation"=w285:enum16{"Update", "Clear"})  [unwired: 1 out]
            n145 = local read "Command Selection"() -> (w284:i32)
            n146 = property on="Command Selection" class="MCListbox (strict)"("ActiveCell"=w292, "CellBG"=w291, "ActiveCell"=w290, "CellBG"=w289) -> ()  [unwired: 2 in, 2 out]
            n147 = call <vilib>:"WPI_DashboardUpdate RPC Info.vi"("Operation"=w285) -> ("update"=w283:bool, "commands"=w282:string[][])  [unwired: 9 in]
            n148 = property on="Command Selection" class="MCListbox (strict)"("ItemNames"=w282) -> ()  [unwired: 2 in, 2 out]
            n149 = property on="Command Params" class="Tbl (strict)"("Active Cell"=w292, "Cell BG Color"=w291, "Active Cell"=w290, "Cell BG Color"=w289) -> ()  [unwired: 2 in, 2 out]
            n150 = call <vilib>:"WPI_DashboardUpdate Command Params.vi"("Update"=w283, "NewVal"=w284, "Commands"=w282, "Param Tbl"=w281) -> ()  [unwired: 7 in, 1 out]
          }
        }
        n151 = call <vilib>:"Connextion Info.vi"() -> ("Connected"=→"NT Connection":bool)  [unwired: 10 in, 1 out]
      }
      event "Test Tree": Value Change {
        # "Show appropriate\ncontrols"
        n152 = event-data() -> ("CtlRef"=w298:refnum<vi>, "NewVal"=w296:string)  [unwired: 1 in]
        n153 = call <vilib>:"WPI_UtilitiesGetTreeIOName.vi"("NewVal"=w296, "TreeControl in"=w298) -> ("I/O Name"=w299:string)  [unwired: 9 in]
        n154 = case shown="\"Camera\"" w299 {
          selector: w299 -> [_ w306 _ w328 w337 _]
          tunnel: w296 -> [_ _ w325 w327 _ w344]
          tunnel: cluster{string[]}[] [{["640x480", "320x240", "160x120"]}, {["Auto", "Fixed indoor", "Fixed outdoor 1", "Fixed outdoor 2", "Fixed fluorescent 1", "Fixed fluorescent 2", "Hold current"]}, {["Auto", "Flicker-free 50 Hz", "Flicker-free 60 Hz", "Hold current"]}, {["None", "Prioritize frame rate", "Prioritize image quality"]}, {["Monochrome", "Color"]}] -> [_ _ _ _ _ w343]
          frame Default {
            w301 = FALSE ("Visible")
            w300 = FALSE ("Visible")
            n155 = property on="Motor" class="Clust (strict)"("Visible"=w300) -> ()  [unwired: 2 in, 2 out]
            n156 = property on="Test Ring" class="Ring (strict)"("Visible"=w300) -> ()  [unwired: 2 in, 2 out]
            n157 = property on="Rev/Fwd" class="Clust (strict)"("Visible"=w301) -> ()  [unwired: 2 in, 2 out]
            n158 = property on="On/Off" class="Bool (strict)"("Visible"=w301) -> ()  [unwired: 2 in, 2 out]
            n159 = property on="Test Slider" class="Slide (strict)"("Visible"=w301) -> ()  [unwired: 2 in, 2 out]
          }
          frame "Analog Out", "Motor", "PWM" {
            w307 = FALSE ("Visible")
            n160 = case shown="\"Analog Out\"" w306 {
              tunnel: [1.0 ("Value") -1.0 ("Value") 0.0 ("Value")] -> w305
              tunnel: [255.0 ("Value") 1.0 ("Value") 5.0 ("Value")] -> w304
              tunnel: [128.0 ("Value") 0.0 ("Value") 0.0 ("Value")] -> w303
              tunnel: [64.0 ("Value") 0.5 ("Value") 1.0 ("Value")] -> w302
              frame "PWM" {
              }
              frame "Motor", Default {
              }
              frame "Analog Out" {
              }
            }
            n161 = property on="Motor" class="Clust (strict)"("Visible"=TRUE) -> ()  [unwired: 2 in, 2 out]
            n162 = property on="Value" class="Slide (strict)"("Value"=w303, "Scale.Minimum"=w305, "Scale.Maximum"=w304, "Scale.Increment"=w302) -> ()  [unwired: 2 in, 2 out]
            n163 = property on="On/Off" class="Bool (strict)"("Visible"=w307) -> ()  [unwired: 2 in, 2 out]
            n164 = property on="Test Slider" class="Slide (strict)"("Visible"=w307) -> ()  [unwired: 2 in, 2 out]
            n165 = property on="Test Ring" class="Ring (strict)"("Visible"=w307) -> ()  [unwired: 2 in, 2 out]
            n166 = property on="Rev/Fwd" class="Clust (strict)"("Visible"=w307) -> ()  [unwired: 2 in, 2 out]
          }
          frame "Servo" {
            w323 = FALSE ("Visible")
            n167 = call <vilib>:"NT Read Number.vi"("Name"=w325) -> ("Numeric"=w324:dbl)  [unwired: 9 in, 1 out]
            n168 = property on="Test Slider" class="Slide (strict)"("Visible"=TRUE, "Scale.Maximum"=170.0 ("Scale.Range:Maximum")) -> ()  [unwired: 2 in, 2 out]
            n169 = local write "Test Slider"(w324) -> ()
            n170 = property on="Motor" class="Clust (strict)"("Visible"=w323) -> ()  [unwired: 2 in, 2 out]
            n171 = property on="Rev/Fwd" class="Clust (strict)"("Visible"=w323) -> ()  [unwired: 2 in, 2 out]
            n172 = property on="On/Off" class="Bool (strict)"("Visible"=w323) -> ()  [unwired: 2 in, 2 out]
            n173 = property on="Test Ring" class="Ring (strict)"("Visible"=w323) -> ()  [unwired: 2 in, 2 out]
          }
          frame "Relay", "Solenoid" {
            w326 = FALSE ("Visible")
            n174 = property on="Motor" class="Clust (strict)"("Visible"=w326) -> ()  [unwired: 2 in, 2 out]
            n175 = property on="Test Slider" class="Slide (strict)"("Visible"=w326) -> ()  [unwired: 2 in, 2 out]
            n176 = Search and Replace String(input string=w327, search string="/Value  **", replace string="/Direction") -> (result string=w333:string)  [unwired: 5 in, 3 out]
            n177 = property on="Test Ring" class="Ring (strict)"("Visible"=w326) -> ()  [unwired: 2 in, 2 out]
            n178 = call <vilib>:"NT Read String.vi"("Name"=w333) -> ("String"=w331:string)  [unwired: 9 in, 1 out]
            n179 = Equal?(x="Both directions", y=w331) -> (x = y?=w329:bool)
            n180 = Not(x=w329) -> (.not. x?=w330:bool)
            n181 = property on="Rev/Fwd" class="Clust (strict)"("Visible"=w329) -> ()  [unwired: 2 in, 2 out]
            n182 = property on="On/Off" class="Bool (strict)"("Visible"=w330, "Caption.Text"=w328) -> ()  [unwired: 2 in, 2 out]
          }
          frame "Compressor", "Digital Out" {
            w336 = FALSE ("Visible")
            # "Get direction and finish"
            n183 = property on="Motor" class="Clust (strict)"("Visible"=w336) -> ()  [unwired: 2 in, 2 out]
            n184 = property on="Test Slider" class="Slide (strict)"("Visible"=w336) -> ()  [unwired: 2 in, 2 out]
            n185 = property on="Test Ring" class="Ring (strict)"("Visible"=w336) -> ()  [unwired: 2 in, 2 out]
            n186 = property on="On/Off" class="Bool (strict)"("Visible"=TRUE, "Caption.Text"=w337) -> ()  [unwired: 2 in, 2 out]
            n187 = property on="Rev/Fwd" class="Clust (strict)"("Visible"=FALSE) -> ()  [unwired: 2 in, 2 out]
          }
          frame "Camera" {
            n188 = call <vilib>:"Get Last Path Segment.vi"("String in"=w344) -> ("String out"=w345:string)  [unwired: 10 in]
            n189 = property on="On/Off" class="Bool (strict)"("Visible"=FALSE) -> ()  [unwired: 2 in, 2 out]
            n190 = property on="Motor" class="Clust (strict)"("Visible"=FALSE) -> ()  [unwired: 2 in, 2 out]
            n191 = property on="Rev/Fwd" class="Clust (strict)"("Visible"=FALSE) -> ()  [unwired: 2 in, 2 out]
            n192 = case shown="\"White Balance  **\"" w345 {
              tunnel: w344 -> [w351 w360 w369 w378 w387 _ w393]
              tunnel: w343 -> [w349 w357 w366 w375 w384 _ _]
              frame "Size  **" {
                n193 = Index Array(array=w349) -> (element=w348:cluster{string[]})  [unwired: 1 in]
                n194 = call <vilib>:"NT Read String.vi"("Name"=w351) -> ("String"=w350:string)  [unwired: 9 in, 1 out]
                n195 = Unbundle(w348) -> (w346:string[])
                n196 = Match First String(2:w346, 3:w350) -> (0:w347:i32)  [unwired: 1 out]
                n197 = property on="Test Ring" class="Ring (strict)"("Value"=w347, "Strings []"=w346) -> ()  [unwired: 2 in, 2 out]
                n198 = property on="Test Ring" class="Ring (strict)"("Visible"=TRUE) -> ()  [unwired: 2 in, 2 out]
                n199 = property on="Test Slider" class="Slide (strict)"("Visible"=FALSE) -> ()  [unwired: 2 in, 2 out]
              }
              frame "White Balance  **" {
                n200 = Index Array(array=w357, index=1) -> (element=w358:cluster{string[]})
                n201 = call <vilib>:"NT Read String.vi"("Name"=w360) -> ("String"=w359:string)  [unwired: 9 in, 1 out]
                n202 = Unbundle(w358) -> (w355:string[])
                n203 = Match First String(2:w355, 3:w359) -> (0:w354:i32)  [unwired: 1 out]
                n204 = property on="Test Ring" class="Ring (strict)"("Value"=w354, "Strings []"=w355) -> ()  [unwired: 2 in, 2 out]
                n205 = property on="Test Ring" class="Ring (strict)"("Visible"=TRUE) -> ()  [unwired: 2 in, 2 out]
                n206 = property on="Test Slider" class="Slide (strict)"("Visible"=FALSE) -> ()  [unwired: 2 in, 2 out]
              }
              frame "Exposure  **" {
                n207 = Index Array(array=w366, index=2) -> (element=w367:cluster{string[]})
                n208 = call <vilib>:"NT Read String.vi"("Name"=w369) -> ("String"=w368:string)  [unwired: 9 in, 1 out]
                n209 = Unbundle(w367) -> (w363:string[])
                n210 = Match First String(2:w363, 3:w368) -> (0:w364:i32)  [unwired: 1 out]
                n211 = property on="Test Ring" class="Ring (strict)"("Value"=w364, "Strings []"=w363) -> ()  [unwired: 2 in, 2 out]
                n212 = property on="Test Ring" class="Ring (strict)"("Visible"=TRUE) -> ()  [unwired: 2 in, 2 out]
                n213 = property on="Test Slider" class="Slide (strict)"("Visible"=FALSE) -> ()  [unwired: 2 in, 2 out]
              }
              frame "Exposure Priority  **" {
                n214 = Index Array(array=w375, index=3) -> (element=w376:cluster{string[]})
                n215 = call <vilib>:"NT Read String.vi"("Name"=w378) -> ("String"=w377:string)  [unwired: 9 in, 1 out]
                n216 = Unbundle(w376) -> (w372:string[])
                n217 = Match First String(2:w372, 3:w377) -> (0:w373:i32)  [unwired: 1 out]
                n218 = property on="Test Ring" class="Ring (strict)"("Value"=w373, "Strings []"=w372) -> ()  [unwired: 2 in, 2 out]
                n219 = property on="Test Ring" class="Ring (strict)"("Visible"=TRUE) -> ()  [unwired: 2 in, 2 out]
                n220 = property on="Test Slider" class="Slide (strict)"("Visible"=FALSE) -> ()  [unwired: 2 in, 2 out]
              }
              frame "Color Enable  **" {
                n221 = Index Array(array=w384, index=4) -> (element=w385:cluster{string[]})
                n222 = call <vilib>:"NT Read String.vi"("Name"=w387) -> ("String"=w386:string)  [unwired: 9 in, 1 out]
                n223 = Unbundle(w385) -> (w381:string[])
                n224 = Match First String(2:w381, 3:w386) -> (0:w382:i32)  [unwired: 1 out]
                n225 = property on="Test Ring" class="Ring (strict)"("Value"=w382, "Strings []"=w381) -> ()  [unwired: 2 in, 2 out]
                n226 = property on="Test Ring" class="Ring (strict)"("Visible"=TRUE) -> ()  [unwired: 2 in, 2 out]
                n227 = property on="Test Slider" class="Slide (strict)"("Visible"=FALSE) -> ()  [unwired: 2 in, 2 out]
              }
              frame Default {
                n228 = property on="Test Ring" class="Ring (strict)"("Visible"=FALSE) -> ()  [unwired: 2 in, 2 out]
                n229 = property on="Test Slider" class="Slide (strict)"("Visible"=FALSE) -> ()  [unwired: 2 in, 2 out]
              }
              frame "Brightness  **", "Color Level  **", "Compression  **", "FPS  **", "Sharpness  **" {
                n230 = call <vilib>:"NT Read Number.vi"("Name"=w393) -> ("Numeric"=w392:dbl)  [unwired: 9 in, 1 out]
                n231 = local write "Test Slider"(w392) -> ()
                n232 = property on="Test Slider" class="Slide (strict)"("Visible"=TRUE, "Scale.Maximum"=100.0 ("Scale.Range:Maximum")) -> ()  [unwired: 2 in, 2 out]
                n233 = property on="Test Ring" class="Ring (strict)"("Visible"=FALSE) -> ()  [unwired: 2 in, 2 out]
              }
            }
          }
        }
        n234 = property on="Progress" class="Clust (strict)"("Visible"=FALSE) -> ()  [unwired: 2 in, 2 out]
      }
      event "Test Name": Mouse Enter {
        # "Populate the ring with the list of tests"
        n235 = event-data() -> ()  [unwired: 1 in, 1 out]
        n236 = call <vilib>:"NT Read String Array.vi"("Name"="/TestMode/TestList") -> ("String Array"=w401:string[])  [unwired: 9 in, 1 out]
        n237 = Build Array (concatenate)("Select the test to run...", w401) -> (w400:string[])
        n238 = property on="Test Name" class="Ring (strict)"("Strings []"=w400) -> ()  [unwired: 2 in, 2 out]
      }
      event "Test Name": Value Change {
        w403 = FALSE ("Visible")
        # "Tell the robot the test name to run"
        n239 = event-data() -> ("NewVal"=w407:u16)  [unwired: 1 in]
        n240 = property on="Test Name" class="Ring (strict)"() -> ("Strings []"=w408:string[])  [unwired: 2 in, 2 out]
        n241 = local write "Progress"(T6 {"Test Progress"=0, "Test Progress Text"=""} ("Progress")) -> ()
        n242 = Index Array(array=w408, index=w407) -> (element=w406:string)
        n243 = call <vilib>:"NT Write String.vi"("String"=w406, "Name"="/TestMode/TestName") -> ()  [unwired: 9 in, 1 out]
        n244 = property on="Progress" class="Clust (strict)"("Visible"=TRUE) -> ()  [unwired: 2 in, 2 out]
        n245 = property on="Motor" class="Clust (strict)"("Visible"=w403) -> ()  [unwired: 2 in, 2 out]
        n246 = property on="Test Slider" class="Slide (strict)"("Visible"=w403) -> ()  [unwired: 2 in, 2 out]
        n247 = property on="On/Off" class="Bool (strict)"("Visible"=w403) -> ()  [unwired: 2 in, 2 out]
        n248 = property on="Rev/Fwd" class="Clust (strict)"("Visible"=w403) -> ()  [unwired: 2 in, 2 out]
        n249 = property on="Test Ring" class="Ring (strict)"("Visible"=w403) -> ()  [unwired: 2 in, 2 out]
      }
      event "Command Selection": Value Change {
        # "Get the params and show in table"
        n250 = event-data() -> ("NewVal"=w413:i32)  [unwired: 1 in]
        n251 = property on="Command Selection" class="MCListbox (strict)"() -> ("ItemNames"=w411:string[][])  [unwired: 2 in, 2 out]
        n252 = call <vilib>:"WPI_DashboardUpdate Command Params.vi"("NewVal"=w413, "Commands"=w411, "Param Tbl"=w412) -> ()  [unwired: 8 in, 1 out]
      }
      event "Execute Command": Value Change {
        # "Started one, Unique ID holds\nresponse"
        n253 = event-data() -> ()  [unwired: 1 in, 1 out]
        n254 = property on="Command Selection" class="MCListbox (strict)"() -> ("ItemNames"=w424:string[][])  [unwired: 2 in, 2 out]
        n255 = Index Array(array=w424, index (row)="Command Selection", index (col)=0) -> (element=w422:string)
        n256 = call <vilib>:"Invoke Commands.vi"("Command Params"="Command Params", "Function Name"=w422) -> ("Params"=w418:u8, "Started"=w417:bool)  [unwired: 7 in, 1 out]
        n257 = Array Subset(array="Command Params", length (row)=w418) -> (w419:string[][])  [unwired: 3 in]
        n258 = Select(t="Executing" ("Cmd Status"), s=w417, f="" ("Cmd Status")) -> (s? t:f=→"Cmd Status":string)
      }
      event "Command Selection": Double Click {
        n259 = event-data() -> ("Row"=w432:i32)  [unwired: 1 in]
        n260 = property on="Command Selection" class="MCListbox (strict)"() -> ("ItemNames"=w435:string[][])  [unwired: 2 in, 2 out]
        n261 = local read "Command Params"() -> (w431:string[][])
        n262 = Index Array(array=w435, index (row)=w432, index (col)=0) -> (element=w433:string)
        n263 = call <vilib>:"Invoke Commands.vi"("Command Params"=w431, "Function Name"=w433) -> ("Params"=w430:u8, "Started"=w425:bool)  [unwired: 7 in, 1 out]
        n264 = Array Subset(array=w431, length (row)=w430) -> (w429:string[][])  [unwired: 3 in]
        n265 = Select(t="Executing" ("Cmd Status"), s=w425, f="" ("Cmd Status")) -> (s? t:f=w426:string)
        n266 = local write "Cmd Status"(w426) -> ()
      }
      event "CheckList": Double Click {
        # "Shift clears all"
        # "Update symbols on the listbox"
        n267 = event-data() -> ("PlatMods.Shift"=w437:bool, "Row"=w439:i32)  [unwired: 1 in]
        n268 = case shown="True" w437 {
          tunnel: w439 -> [w443 _]
          tunnel: 1 -> [w442 _]
          frame False {
            n269 = property on="CheckList" class="LstBox (strict)"() -> ("Item Symbols"=w441:i32[])  [unwired: 2 in, 2 out]
            n270 = Replace Array Subset(array=w441, new element=w442, index=w443) -> (w440:i32[])
            n271 = property on="CheckList" class="LstBox (strict)"("Item Symbols"=w440) -> ()  [unwired: 2 in, 2 out]
          }
          frame True {
            w444 = 0 ("Top Row")
            n272 = property on="CheckList" class="LstBox (strict)"() -> ("Number of Rows"=w446:u32)  [unwired: 2 in, 2 out]
            n273 = Initialize Array(0, w446) -> (w445:i32[])
            n274 = property on="CheckList" class="LstBox (strict)"("Top Row"=w444, "Value"=w444, "Item Symbols"=w445) -> ()  [unwired: 2 in, 2 out]
          }
        }
      }
      event "CheckList": Key Down {
        # "Update symbols on the listbox\nLeft and right keys check and uncheck"
        n275 = event-data() -> ("VKey"=w450:T20)  [unwired: 1 in]
        n276 = case shown="\"Left\", \"Right\"" w450 {
          selector: w450 -> [w455 _]
          tunnel: eventvkey."Left" ("VKey") -> [w453 _]
          frame "Left", "Right" {
            n277 = Equal?(x=w453, y=w455) -> (x = y?=w454:bool)
            n278 = Select(t=0, s=w454, f=1) -> (s? t:f=w456:i32)
            n279 = property on="CheckList" class="LstBox (strict)"() -> ("Item Symbols"=w459:i32[])  [unwired: 2 in, 2 out]
            n280 = Replace Array Subset(array=w459, new element=w456, index="CheckList") -> (w458:i32[])
            n281 = property on="CheckList" class="LstBox (strict)"("Item Symbols"=w458) -> ()  [unwired: 2 in, 2 out]
          }
          frame Default {
          }
        }
      }
      event "Motor.Enable": Value Change {
        # "When the test mode otor enable helper is set, update that\ntree row item's value"
        n282 = event-data() -> ("NewVal"=w465:bool)  [unwired: 1 in]
        n283 = Unbundle("Motor") -> ("Value"=w464:dbl)  [unwired: 1 out]
        n284 = Select(t=w464, s=w465, f=0.0) -> (s? t:f=w462:dbl)
        n285 = call <vilib>:"NT Write Number.vi"("Numeric"=w462, "Name"=w461) -> ()  [unwired: 9 in, 1 out]
      }
      event "Test Slider": Value Change {
        # "When the test mode slider helper is set, update that\ntree row item's value"
        n286 = event-data() -> ("NewVal"=w468:dbl)  [unwired: 1 in]
        n287 = call <vilib>:"NT Write Number.vi"("Numeric"=w468, "Name"=w469) -> ()  [unwired: 9 in, 1 out]
      }
      event "On/Off": Value Change {
        # "When the test mode on/off helper value is set, update that\ntree row item's value"
        n288 = event-data() -> ("NewVal"=w473:bool)  [unwired: 1 in]
        n289 = Boolean To (0,1)(Boolean=w473) -> (0, 1=w472:i16)
        n290 = call <vilib>:"NT Write Number.vi"("Numeric"=w472, "Name"=w471) -> ()  [unwired: 9 in, 1 out]
      }
      event "Rev/Fwd": Value Change {
        # "When the test mode helper value for relays is set, update that\ntree row item's value"
        n291 = event-data() -> ("NewVal.Forward"=w481:bool, "NewVal.Reverse"=w480:bool)  [unwired: 1 in]
        n292 = Boolean To (0,1)(Boolean=w481) -> (0, 1=w477:i16)
        n293 = Boolean To (0,1)(Boolean=w480) -> (0, 1=w479:i16)
        n294 = Negate(x=w479) -> (-x=w478:i16)
        n295 = Add(x=w477, y=w478) -> (x+y=w476:i16)
        n296 = call <vilib>:"NT Write Number.vi"("Numeric"=w476, "Name"=w475) -> ()  [unwired: 9 in, 1 out]
      }
      event "Test Ring": Value Change {
        # "When a test mode helper value is selected from the ring,\nset the tree item's variable to the string value"
        n297 = event-data() -> ("NewVal"=w485:u16)  [unwired: 1 in]
        n298 = property on="Test Ring" class="Ring (strict)"() -> ("Strings []"=w486:string[])  [unwired: 2 in, 2 out]
        n299 = Index Array(array=w486, index=w485) -> (element=w484:string)
        n300 = call <vilib>:"NT Write String.vi"("String"=w484, "Name"=w483) -> ()  [unwired: 9 in, 1 out]
      }
      event "Rec Mode": Value Change {
        # "Update globals for recording mode and path to read log from.\nClear when logging and let NetworkTables set path for vision to\nuse."
        n301 = event-data() -> ("NewVal"=w497:enum32{"Stop", "Record", "Playback"})  [unwired: 1 in]
        n302 = global write "WPI_DashboardLogging Global.vi" "Logging Filename"(path "") -> ()
        n303 = global write "WPI_DashboardLogging Global.vi" "Recording"(w497) -> ()
        n304 = case shown="\"Playback\"" w497 {
          tunnel: w496 -> [_ w499 w508]
          tunnel: [_ _ w507] -> w494
          tunnel: [_ _ w506] -> _
          tunnel: w492 -> [_ _ w504]
          tunnel: cluster{i32, i32} {-250, 170} -> [_ _ w503]
          tunnel: [_ _ T21 {"Image Size"=TRUE, "Image Type"=TRUE, "Pixel Value"=TRUE, "ROI Information"=TRUE, "Zoom Factor"=FALSE} ("Image Information Shown:All Elements")] -> w490
          tunnel: [_ _ TRUE ("Zoom Factor")] -> w489
          tunnel: w488 -> [_ _ w500]
          frame Default {
          }
          frame "Stop", "Record" {
            # "Place Window too"
            n305 = invoke class="VI" method="FP.Close"(reference=w499) -> (reference out=w498:refnum<vi>)  [unwired: 2 in, 2 out]
            n306 = invoke class="VI" method="Abort VI"(reference=w498) -> ()  [unwired: 2 in, 3 out]
          }
          frame "Playback" {
            n307 = call "Open Playback Panel.vi"("Offset"=w503, "DB VI Ref"=w504, "Playback in"=w508) -> ("Playback out"=w505:refnum<vi>)  [unwired: 8 in]
            n308 = register-events(w505, w500) -> (reference out=w507:refnum<event-registration>, error out=w506:errorcluster)  [unwired: 2 in]
          }
        }
        n309 = property on="Camera Image" class="ImageControl"("Image Information Shown"=w490, "Image Information Visible"=w489) -> ()  [unwired: 2 in, 2 out]
        n310 = call <vilib>:"WPI_DashboardNT Log FieldName Cache.vi"("Operation"=enum16{"Lookup/Add", "Index", "Clear"}."Clear") -> ()  [unwired: 8 in, 3 out]
      }
      event Panel Close {
        w510 = enum32{"Stop", "Record", "Playback"}."Stop" ("Rec Mode")
        # "Playback window has been closed, abort"
        n311 = event-data() -> ()  [unwired: 1 in, 4 out]
        n312 = local write "Rec Mode"(w510) -> ()
        n313 = global write "WPI_DashboardLogging Global.vi" "Recording"(w510) -> ()
      }
      event Panel Close {
        # "Abort playback window and ourself"
        n314 = event-data() -> ()  [unwired: 1 in, 4 out]
        n315 = invoke class="VI" method="FP.Close"(reference=w514) -> (reference out=w513:refnum<vi>)  [unwired: 2 in, 2 out]
        n316 = invoke class="VI" method="Abort VI"(reference=w513) -> (error out=w512:errorcluster)  [unwired: 2 in, 2 out]
        n317 = invoke class="VI" method="Abort VI"(error in=w512) -> ()  [unwired: 2 in, 3 out]
      }
      event User Event {
        n318 = event-data() -> ("IDs"=w521:cluster{"RPC field ID":u16, "Unique ID":u16}, "String"=w520:string)  [unwired: 1 in]
        n319 = Bundle("IDs"=w521, "String"=w520) -> (w519:T8)  [unwired: 1 in]
        n320 = call <vilib>:"Retrieve RPC Response.vi"("RPC Response"=w519) -> ("Output"=w517:string[][])  [unwired: 10 in]
        n321 = Build Array (concatenate)(w515, w517) -> (w516:string[][])
        n322 = local write "Command Params"(w516) -> ()
        n323 = local write "Cmd Status"("" ("Cmd Status")) -> ()
      }
      event "Tree": Double Click {
        n324 = event-data() -> ("PlatMods"=w525:T24, "Tag"=w524:string)  [unwired: 1 in]
        n325 = Unbundle(w525) -> ("Shift"=w523:bool)  [unwired: 4 out]
        n326 = Not(x=w523) -> (.not. x?=w522:bool)
        n327 = call <vilib>:"NT Update Persistence.vi"("Persistence"=w522, "Name"=w524) -> ()  [unwired: 9 in, 1 out]
      }
    }
  }
  n328 = while {
    tunnel: w62 -> [w528]
    i -> [w531]
    stop <- FALSE stop-if-true
    n329 = Wait (ms)(milliseconds to wait=u32 100) -> ()  [unwired: 1 out]
    n330 = case shown="\"Playback\"" "Rec Mode" {
      tunnel: w531 -> [_ _ w546]
      tunnel: [u32 2829099 ("Base Color") u32 11141120 ("Target Color") w535] -> w527
      frame "Stop", Default {
        # "Reset the color, extra updates don't cost much"
      }
      frame "Record" {
      }
      frame "Playback" {
        # "Playback"
        n331 = Quotient & Remainder(x=w546, y=u32 50 ("milliseconds to wait")) -> (x-y*floor(x/y)=w542:u32)  [unwired: 1 out]
        n332 = Divide(x=w542, y=u32 50 ("milliseconds to wait")) -> (x/y=w539:dbl)
        n333 = Multiply(x=6.283185307179586, y=w539) -> (x*y=w544:dbl)
        n334 = Sine(x=w544) -> (sin(x)=w543:dbl)
        n335 = Absolute Value(x=w543) -> (abs(x)=w536:dbl)
        n336 = call "Interpolate RGB Color.vi"("Proportion"=w536, "Target Color"=u32 30976, "Base Color"=u32 2829099) -> ("Result Color"=w535:u32)  [unwired: 8 in]
      }
    }
    n337 = property class="Pane"(reference=w528, "PaneColor"=w527) -> ()  [unwired: 1 in, 2 out]
  }
  n338 = local write "Dashboard Tab"(T3."Drive" ("Dashboard Tab")) -> ()
  n339 = property on="On/Off" class="Bool (strict)"("Visible"=w31) -> ()  [unwired: 2 in, 2 out]
  n340 = property on="Motor" class="Clust (strict)"("Visible"=w31) -> ()  [unwired: 2 in, 2 out]
  n341 = property on="Progress" class="Clust (strict)"("Visible"=w31) -> ()  [unwired: 2 in, 2 out]
  n342 = property on="Test Ring" class="Ring (strict)"("Visible"=w31) -> ()  [unwired: 2 in, 2 out]
  n343 = property on="Rev/Fwd" class="Clust (strict)"("Visible"=w31) -> ()  [unwired: 2 in, 2 out]
  n344 = while {
    tunnel: u16 1741 ("timeout ms (25000)") -> [w548]
    stop <- FALSE stop-if-true
    n345 = TCP Create Listener(10:w548) -> (0:w547:errorcluster, 3:w549:refnum<k5>)  [unwired: 4 in, 1 out]
    n346 = case shown="No Error" w547 {
      selector: w547 -> [w551 _]
      tunnel: w549 -> [w552 _]
      frame No Error {
        n347 = while {
          tunnel: w552 -> [w555]
          tunnel: w551 -> [w554]
          stop <- FALSE stop-if-true
          n348 = TCP Wait On Listener(8:w554, 11:w555) -> (0:w556:errorcluster, 4:w557:refnum<k5>)  [unwired: 2 in, 3 out]
          n349 = local write "TCP"(w557) -> ()
          n350 = case shown="No Error" w556 {
            frame No Error {
            }
            frame Error {
              n351 = Wait (ms)(milliseconds to wait=u32 1000) -> ()  [unwired: 1 out]
            }
          }
        }
      }
      frame Error {
        n352 = Wait (ms)(milliseconds to wait=u32 1000) -> ()  [unwired: 1 out]
      }
    }
  }
  n353 = local write "Command Selection"(u16 0 ("milliseconds to wait")) -> ()
  n354 = local write "Command Params"(string[][] [] ("Command Params")) -> ()
  n355 = global write "WPI_DashboardLogging Global.vi" "Recording"(w56) -> ()
  n356 = local write "Rec Mode"(w56) -> ()
